vi "File.CSV, Write Name Value, String.vi"(8 "error in":errorcluster, 9 "New Val":string[](array[string]), 10 "Names":string[](array[string]), 11 "CSV File":path) -> (0 "error out":errorcluster, 1 "Values Out":string[](array[string]), 2 "Names Out":string[](array[string]), 3 "Changed":bool)   [LabVIEW 2024]
uses:
  <vilib>/KATE/Files/File Utils.lvlib
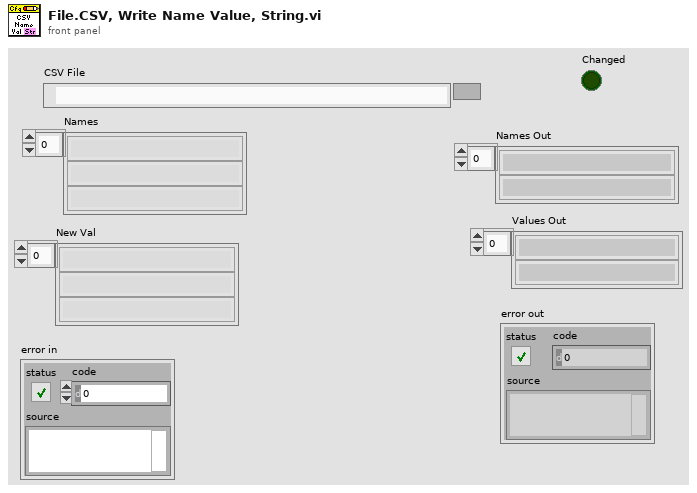
[diagram p1: front panel]
types:
  T1 = enum16{"open", "replace", "create", "open or create", "replace or create", "replace or create with confirmation"}
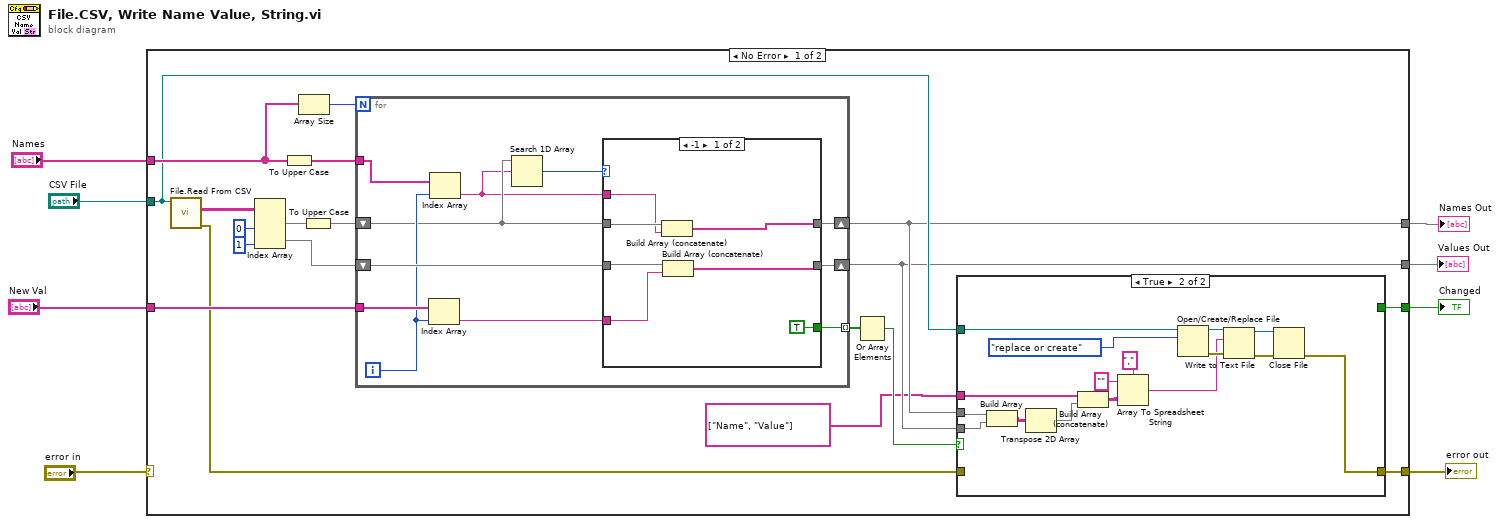
[diagram p0: block diagram]
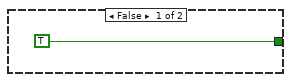
[diagram p2: hidden frame]
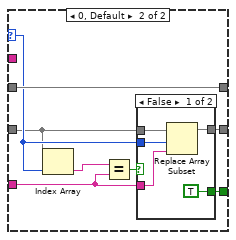
[diagram p3: hidden frame]
diagram:
  n1 = case shown="No Error" "error in" {
    selector: "error in" -> [_ w79]
    tunnel: "CSV File" -> [w16 _]
    tunnel: "New Val" -> [w18 w77]
    tunnel: "Names" -> [w21 w78]
    tunnel: [w15 w78] -> w6
    tunnel: [w14 w77] -> w5
    tunnel: [w10 w79] -> w3
    tunnel: [w13 _] -> w1
    frame No Error {
      n2 = call <vilib>:"File.Read From CSV.vi"("File"=w16) -> ("error out"=w12:errorcluster, "Data"=w27:string[][])  [unwired: 8 in, 1 out]
      n3 = Index Array(array=w27, index (col) #1=0 ("disabled index (col)"), index (col) #2=1 ("index (col)")) -> (element #1=w24:string[], element #2=w19:string[])  [unwired: 2 in]
      n4 = To Upper Case(1:w21) -> (0:w23:string[])
      n5 = Array Size(array=w21) -> (size(s)=w20:i32)
      n6 = To Upper Case(1:w24) -> (0:w22:string[])
      n7 = for {
        N: w20 -> [_]
        tunnel: w18 -> [w52]
        tunnel: w23 -> [w47]
        shift-right: [w50] -> w15
        shift-left: w22 -> [w46]
        shift-right: [w53] -> w14
        shift-left: w19 -> [w54]
        tunnel: [w48] -> w17 mode=indexing
        i -> [w51]
        n8 = Index Array(array=w52, index=w51) -> (element=w49:string)
        n9 = Index Array(array=w47, index=w51) -> (element=w45:string)
        n10 = Search 1D Array(1D array=w46, element=w45) -> (index of element=w55:i32)  [unwired: 1 in]
        n11 = case shown="-1" w55 {
          selector: w55 -> [_ w68]
          tunnel: w54 -> [w59 w67]
          tunnel: [w57 w70] -> w53
          tunnel: w49 -> [w58 w65]
          tunnel: w46 -> [w62 w69]
          tunnel: [w61 w69] -> w50
          tunnel: w45 -> [w60 _]
          tunnel: [TRUE w63] -> w48
          frame -1 {
            n12 = Build Array (concatenate)(w62, w60) -> (w61:string[])
            n13 = Build Array (concatenate)(w59, w58) -> (w57:string[])
          }
          frame 0, Default {
            n14 = Index Array(array=w67, index=w68) -> (element=w66:string)
            n15 = Equal?(x=w66, y=w65) -> (x = y?=w64:bool)
            n16 = case shown="False" w64 {
              tunnel: [w75 w76] -> w70
              tunnel: w68 -> [w74 _]
              tunnel: w67 -> [w73 w76]
              tunnel: w65 -> [w72 _]
              tunnel: [TRUE _] -> w63
              frame False {
                n17 = Replace Array Subset(array=w73, new element=w72, index=w74) -> (w75:string[])
              }
              frame True {
              }
            }
          }
        }
      }
      n18 = Or Array Elements(Boolean array=w17) -> (logical OR=w11:bool)
      n19 = case shown="True" w11 {
        tunnel: w16 -> [_ w35]
        tunnel: w15 -> [_ w43]
        tunnel: w14 -> [_ w42]
        tunnel: string[] ["Name", "Value"] -> [_ w44]
        tunnel: [TRUE _] -> w13
        tunnel: w12 -> [_ _]
        tunnel: [_ w31] -> w10
        frame False {
        }
        frame True {
          n20 = Build Array(w43, w42) -> (w41:string[][])
          n21 = Transpose 2D Array(2D array=w41) -> (transposed array=w40:string[][])
          n22 = Build Array (concatenate)(w44, w40) -> (w39:string[][])
          n23 = Array To Spreadsheet String(delimiter (Tab)=",", array=w39, 3:"" ("format string")) -> (spreadsheet string=w30:string)
          n24 = Open/Create/Replace File(file path (use dialog)=w35, operation (0:open)=T1."replace or create") -> (refnum out=w34:refnum<file>, error out=w36:errorcluster)  [unwired: 4 in, 1 out]
          n25 = Write to Text File(file (use dialog)=w34, text=w30, error in=w36) -> (refnum out=w32:refnum<file>, error out=w33:errorcluster)  [unwired: 1 in, 1 out]
          n26 = Close File(refnum=w32, error in=w33) -> (error out=w31:errorcluster)  [unwired: 1 out]
        }
      }
    }
    frame Error {
    }
  }
  "Values Out" <- w5
  "Names Out" <- w6
  "error out" <- w3
  "Changed" <- w1
